vi "subvi v to p.vi"() -> ()   [LabVIEW 2016]
panel:
  in  "stop":bool
  out "Output Variable 2":dbl format="%#_3e"
  out "output variable 3":dbl format="%#_3e"
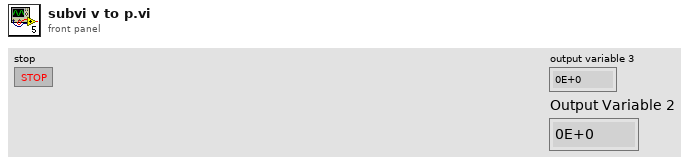
[diagram p1: front panel]
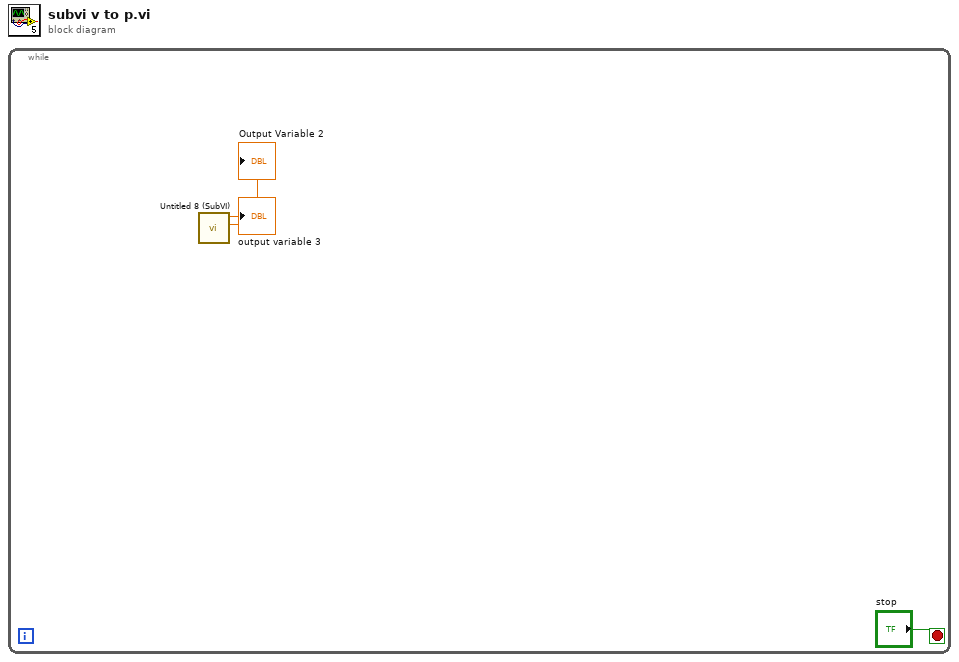
[diagram p0: block diagram]
diagram:
  n1 = while {
    stop <- "stop" stop-if-true
    n2 = call "Untitled 8 (SubVI).vi"() -> ("Output Variable 2"=→"Output Variable 2":dbl, "output variable 3"=→"output variable 3":dbl)  [unwired: 10 in]
  }
